vi "Scanned Write - UDV.vi"(5 "FXP VI Ref":refnum<vi>, 7 "UDV Data Type":T2, 8 "error in (no error)":errorcluster, 9 "FXP Config":T1, 10 "data in":dbl, 11 "IOV ref in":refnum<k21>) -> (0 "error out":errorcluster, 3 "IOV ref out":refnum<k21>)   [LabVIEW 2017, in "Scan Engine Custom Device.lvlib"]
uses:
  Scan Engine Custom Device.lvlib
  Type Defs/UDV Data Type.ctl
  Type Defs/FXP Config.ctl
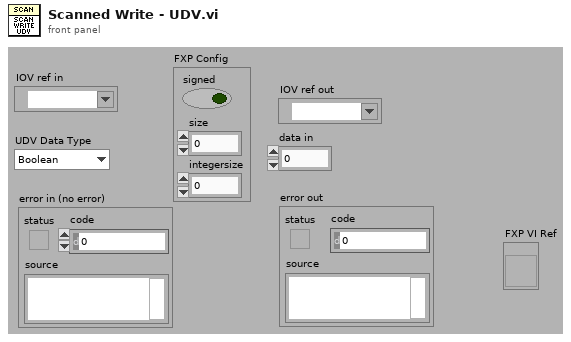
[diagram p1: front panel]
types:
  T1 = typedef "Scan Engine Custom Device.lvlib/FXP Config.ctl" = cluster{"signed":bool, "size":u32, "integersize":i32}
  T2 = typedef "Scan Engine Custom Device.lvlib/UDV Data Type.ctl" = enum16{"Boolean", "Fixed Point", "Int8", "Int16", "Int32", "Int64", "U32 Bit Field", "UInt8", "UInt16", "UInt32", "UInt64", "Other"}
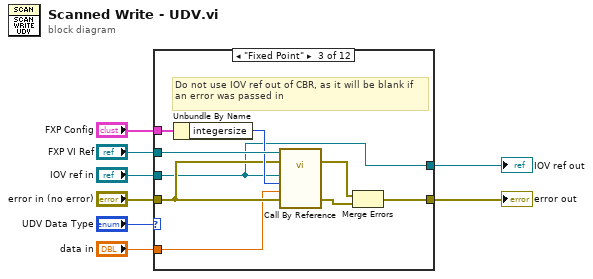
[diagram p0: block diagram]
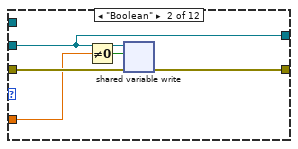
[diagram p3: hidden frame]
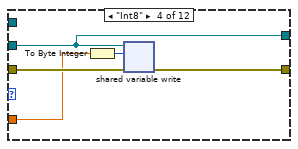
[diagram p4: hidden frame]
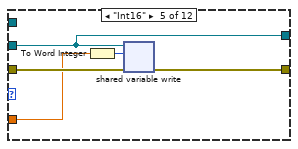
[diagram p5: hidden frame]
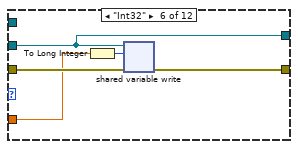
[diagram p6: hidden frame]
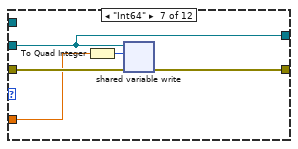
[diagram p7: hidden frame]
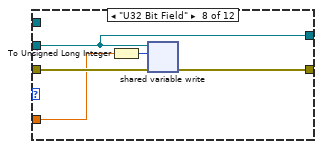
[diagram p8: hidden frame]
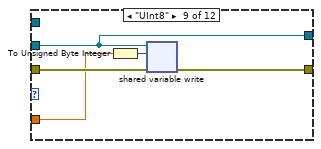
[diagram p9: hidden frame]
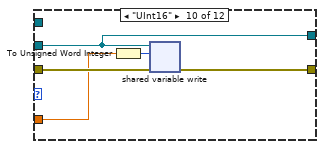
[diagram p10: hidden frame]
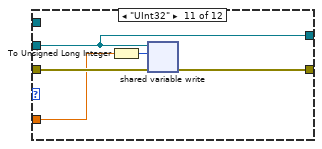
[diagram p11: hidden frame]
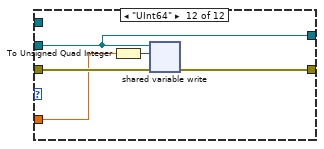
[diagram p12: hidden frame]
diagram:
  n1 = case shown="\"Fixed Point\"" "UDV Data Type" {
    tunnel: "IOV ref in" -> [w10 w13 w16 w27 w32 w37 w42 w47 w52 w57 w62 w67]
    tunnel: [w10 w13 w16 w27 w32 w37 w42 w47 w52 w57 w62 w67] -> w6
    tunnel: "error in (no error)" -> [w9 w15 w21 w29 w34 w39 w44 w49 w54 w59 w64 w69]
    tunnel: [w9 w14 w20 w28 w33 w38 w43 w48 w53 w58 w63 w68] -> w4
    tunnel: "FXP Config" -> [_ _ w23 _ _ _ _ _ _ _ _ _]
    tunnel: "FXP VI Ref" -> [_ _ w24 _ _ _ _ _ _ _ _ _]
    tunnel: "data in" -> [_ w11 w17 w25 w30 w35 w40 w45 w50 w55 w60 w65]
    frame Default {
    }
    frame "Boolean" {
      n2 = Not Equal To 0?(x=w11) -> (x != 0?=w12:bool)
      n3 = shared-variable-write(w13, w15, w12) -> (w14:errorcluster)  [unwired: 1 out]
    }
    frame "Fixed Point" {
      # "Do not use IOV ref out of CBR, as it will be blank if an error was passed in"
      n4 = Unbundle By Name(w23) -> ("integersize"=w22:i32)
      n5 = call-by-ref "?"(reference=w24, error in=w21, 8:"error in (no error)"=w21, "data in"=w17, "integersize"=w22, "shared variable refnum in"=w16) -> (error out=w18:errorcluster, 0:"error out"=w19:errorcluster)  [unwired: 5 in, 3 out]
      n6 = Merge Errors(w18, w19) -> (w20:errorcluster)
    }
    frame "Int8" {
      n7 = To Byte Integer(number=w25) -> (8bit integer=w26:i8)
      n8 = shared-variable-write(w27, w29, w26) -> (w28:errorcluster)  [unwired: 1 out]
    }
    frame "Int16" {
      n9 = To Word Integer(number=w30) -> (16bit integer=w31:i16)
      n10 = shared-variable-write(w32, w34, w31) -> (w33:errorcluster)  [unwired: 1 out]
    }
    frame "Int32" {
      n11 = To Long Integer(number=w35) -> (32bit integer=w36:i32)
      n12 = shared-variable-write(w37, w39, w36) -> (w38:errorcluster)  [unwired: 1 out]
    }
    frame "Int64" {
      n13 = To Quad Integer(1:w40) -> (0:w41:i64)
      n14 = shared-variable-write(w42, w44, w41) -> (w43:errorcluster)  [unwired: 1 out]
    }
    frame "U32 Bit Field" {
      n15 = To Unsigned Long Integer(number=w45) -> (unsigned 32bit integer=w46:u32)
      n16 = shared-variable-write(w47, w49, w46) -> (w48:errorcluster)  [unwired: 1 out]
    }
    frame "UInt8" {
      n17 = To Unsigned Byte Integer(number=w50) -> (unsigned 8bit integer=w51:u8)
      n18 = shared-variable-write(w52, w54, w51) -> (w53:errorcluster)  [unwired: 1 out]
    }
    frame "UInt16" {
      n19 = To Unsigned Word Integer(number=w55) -> (unsigned 16bit integer=w56:u16)
      n20 = shared-variable-write(w57, w59, w56) -> (w58:errorcluster)  [unwired: 1 out]
    }
    frame "UInt32" {
      n21 = To Unsigned Long Integer(number=w60) -> (unsigned 32bit integer=w61:u32)
      n22 = shared-variable-write(w62, w64, w61) -> (w63:errorcluster)  [unwired: 1 out]
    }
    frame "UInt64" {
      n23 = To Unsigned Quad Integer(1:w65) -> (0:w66:u64)
      n24 = shared-variable-write(w67, w69, w66) -> (w68:errorcluster)  [unwired: 1 out]
    }
  }
  "error out" <- w4
  "IOV ref out" <- w6
